vi "Focus judje.vi"(8 "error in":errorcluster, 9 "Standard Variation Limit":sgl, 10 "File Path":path=path "C:/BeamViewImage/TESTIMAGE.png", 11 "Beam Profiler in":refnum<class "Beam Profiler.lvclass">) -> (0 "error out":errorcluster, 2 "Beam Profiler out":refnum<class "Beam Profiler.lvclass">, 3 "离焦？":bool)   [LabVIEW 2018]
uses:
  <instrlib>/nLight Instruments/Beam Profiler/Beam Profiler.lvclass
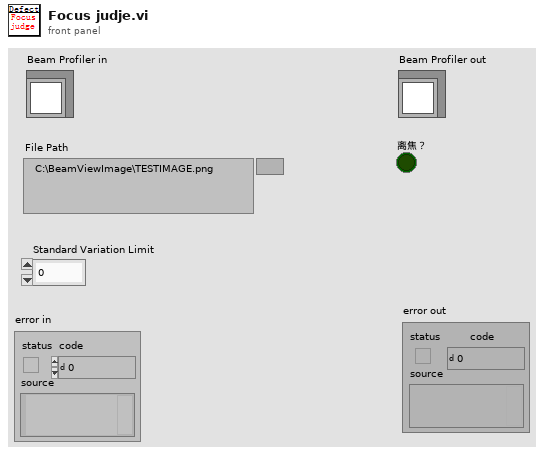
[diagram p1: front panel]
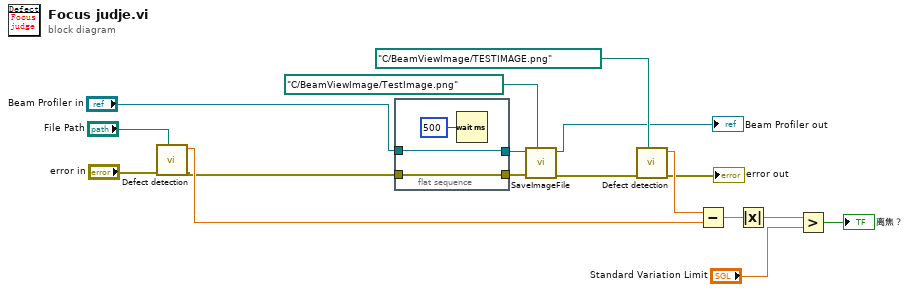
[diagram p0: block diagram]
diagram:
  n1 = call "Defect detection.vi"("File Path"="File Path", "error in"="error in") -> ("error out"=w3:errorcluster, "Standard Variation"=w11:sgl)  [unwired: 8 in]
  n2 = flat-sequence {
    tunnel: w3 -> [w19]
    tunnel: "Beam Profiler in" -> [w18]
    tunnel: [w19] -> w5
    tunnel: [w18] -> w4
    frame #0 {
      n3 = Wait (ms)(milliseconds to wait=u32 500 ("等待时间（毫秒）")) -> ()  [unwired: 1 out]
    }
  }
  n4 = call-dynamic "SaveImageFile.vi"("Path"=path "C:/BeamViewImage/TestImage.png", "error in (no error)"=w5, "Beam Profiler in"=w4) -> ("error out"=w15:errorcluster, "Beam Profiler out"=→"Beam Profiler out":refnum<class "Beam Profiler.lvclass">)  [unwired: 7 in]
  n5 = call "Defect detection.vi"("File Path"=path "C:/BeamViewImage/TESTIMAGE.png", "error in"=w15) -> ("error out"=→"error out":errorcluster, "Standard Variation"=w13:sgl)  [unwired: 8 in]
  n6 = Subtract(x=w13, y=w11) -> (x-y=w10:sgl)
  n7 = Absolute Value(x=w10) -> (abs(x)=w9:sgl)
  n8 = Greater?(x=w9, y="Standard Variation Limit") -> (0:→"离焦？":bool)
